vi "AlliGator Update Settings & Control.vi"(7 "Control Label":string, 8 "Error In":errorcluster, 9 "Value":variant, 10 "Sender":string="AlliGator", 11 "CtlRef":refnum<vi>) -> (0 "Error Out":errorcluster)   [LabVIEW 2021, in "AlliGator Settings.lvlib"]
doc: "Updates the Control whose reference or label is passed.\nThe Settings window is updated as well (or if the Settings Window is the sender, AlliGator is)."
uses:
  AlliGator Settings.lvlib
  AlliGator Settings Event.ctl
  AlliGator Settings Window Messages.ctl
  AlliGator Settings List.ctl
  <vilib>/Utility/error.llb/Error Cluster From Error Code.vi
  Variant/Variant to Data/Variant to Boolean.vi
  <vilib>/ErrorRing/Error Ring.xnode
  Variant/Variant to Data/Variant to Data.lvlib
  Notebook/Notebook.lvlib
  Rich Text Box/Rich Text Box.lvlib
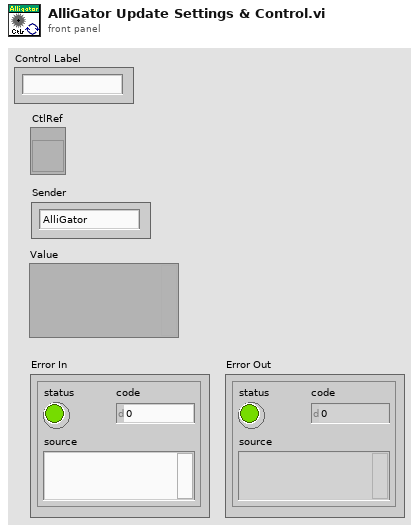
[diagram p1: front panel]
types:
  T1 = typedef "AlliGator Settings.lvlib/AlliGator Settings List.ctl" = enum16{"GUI:Visible Settings Tab", "GUI:Last Run Version", "Source Image:Use Image Histogram for Contrast", "Source Image:Low Count Pixels Rejection Options", "Source Image:High Count Pixels Rejection Options", "Source Image:Use Image Brightness", "Source Image:Blend Overlay with Image Background", "Source Image:Use Fixed ROI Diameter", "Source Image:ROI Diameter", "Source Image:ROI Center Color", "Source Image:Peak Threshold", "Source Image:Intensity Threshold", "Source Image:Image Binning Options", "Source Image:Image Smoothing Options", "Source Image:Image Histogram Active", "Source Image:Invert Binary Mask", "Source Image:Hot Pixel Removal", "Source Image:Overlay Analyzed ROI Center", "Source Image:Auto-Adjust Contrast", "Source Image:Histogram Lower Percentile", "Source Image:Histogram Upper Percentile", "Source Image:Save Source Image", "Source Image:Scale Bar Options", "Source Image:Image Resolution (Pixel Size)", "Source Image:Flatfield Correction", "Source Image:Show Dead Left Columns Correction", "Source Image:Dead Left Columns Correction", "Source Image:Image Pre-Processing Operations Order", "Source Image:Overlay ROI Median", "Source Image:Median Overlay Color", "Data Information:Gate Width", "Data Information:Nanotime Gate Separation", "Data Information:Macrotime Gate Separation", "Data Information:Gate Step", "Data Information:# Gates", "Data Information:Gate Image Exposure", "Data Information:Gate Image Integration", "Data Information:Gates to Skip", "Data Information:Gates to Keep", "Data Information:Define Gates to", "Data Information:Channel Name", "Data Information:Available Channel Names", "Data Information:Channel Arithmetic", "Data Information:Background File Subtraction", "Data Information:Background File", "Data Information:Background Scaling Factor", "Data Information:Background Pile-up Correction", "Data Information:Background Pixel Well Capacity", "Data Information:Laser Period", "Data Information:SYNC Period", "Data Information:Pile-up Correction", "Data Information:Pixel Well Capacity", "Data Information:Dataset Scaling Factor", "Fluorescence Decay_Decay Pre-Processing:Reverse Gates", "Fluorescence Decay_Decay Pre-Processing:Verbose Decay Pre-Processing", "Fluorescence Decay_Decay Pre-Processing:Use Decay Pre-Processing", "Fluorescence Decay_Decay Pre-Processing:Background Subtraction", "Fluorescence Decay_Decay Pre-Processing:Background Definition Range", "Fluorescence Decay_Decay Pre-Processing:Baseline Subtraction Method", "Fluorescence Decay_Decay Pre-Processing:Decay Pre-Processing Operations Order", "Fluorescence Decay_Decay Pre-Processing:Smoothing Parameter", "Fluorescence Decay_Decay Pre-Processing:Shift Decay", "Fluorescence Decay_Decay Pre-Processing:Decay Shift Parameters", "Fluorescence Decay_Decay Pre-Processing:Fold Decay", "Fluorescence Decay_Decay Pre-Processing:# Folds", "Fluorescence Decay_Decay Pre-Processing:1-Normalize Decay", "Fluorescence Decay_Decay Pre-Processing:[0-1]-Normalize Decay", "Fluorescence Decay_Decay Pre-Processing:Smoothen Decay", "Fluorescence Decay_Decay Pre-Processing:Extrapolate Decay", "Fluorescence Decay_Decay Pre-Processing:Use Periodicity", "Fluorescence Decay_Decay Pre-Processing:Use Cursors", "Fluorescence Decay_Decay Pre-Processing:Tail Fraction", "Fluorescence Decay_Decay Pre-Processing:Head Fraction", "Fluorescence Decay_Decay Pre-Processing:Additional Points", "Fluorescence Decay_Decay Pre-Processing:Straighten Decay", "Fluorescence Decay_Decay Pre-Processing:Constant Background", "Fluorescence Decay_Decay Pre-Processing:Pixel-Normalize Decay", "Fluorescence Decay_Advanced Analysis:Extract IRF instead of Decay", "Fluorescence Decay_Advanced Analysis:IRF Extraction Options", "Fluorescence Decay_Advanced Analysis:IRF Optimization Options", "Fluorescence Decay_Advanced Analysis:Square Pulse Options", "Fluorescence Decay_Advanced Analysis:IRF Order", "Fluorescence Decay_Advanced Analysis:IRF Time Constants", "Fluorescence Decay_Advanced Analysis:Wavelet Analysis Options", "Fluorescence Decay_Advanced Analysis:Average Lifetime Options", "Fluorescence Decay_Fit Options:Fit Options", "Fluorescence Decay_Fit Options:Use Legacy Fitting Approach", "Fluorescence Decay_Fit Options:Use Data Information Laser Period", "Fluorescence Decay_Fit Parameters:Displayed Fit Parameters", "Fluorescence Decay_Fit Parameters:Fit Parameter Constraints", "Fluorescence Decay_Fit Parameters:Export Tabulated Results", "Fluorescence Decay_Fit Parameters:MLE Baseline Offset Type", "Fluorescence Decay_Fit Parameters:MLE Baseline Offset", "Fluorescence Decay_Fit Parameters:Guess Parameter Names", "Fluorescence Decay_Fit Parameters:Guess Parameter Values", "Fluorescence Decay_Fit Parameters:Guess Parameters Options", "Fluorescence Decay_Styles:Show Last Decay Only", "Fluorescence Decay_Styles:Decay Graph Color Array", "Fluorescence Decay:Decay Graph Active", "Fluorescence Decay Statistics:Min Peak Value", "Fluorescence Decay Statistics:Reject Low Decay Peak Pixels", "Fluorescence Decay Statistics:Reject High Decay Peak Pixels", "Fluorescence Decay Statistics:Max Peak Value", "Time Traces:Use File Timestamp", "Time Traces:Time Step", "Time Traces:Use Intensity Correction File", "Time Traces:Intensity Correction File", "Phasor Plot:Phasor Plot Smoothing Options", "Phasor Plot:Phasor Plot Size", "Phasor Plot:Phasor Plot Graphics Options", "Phasor Plot:Cumulative Phasor Plot", "Phasor Plot:Use Phasor Brightness", "Phasor Plot:Blend Overlay with Phasor Background", "Phasor Plot:Save Phasor Plot", "Phasor Plot:Show References", "Phasor Plot:Phasor Ratio Decay Range", "Phasor Plot:Exponential Fading", "Phasor Plot:Phasor Ratio Reference Colors", "Phasor Plot:Reference Radius", "Phasor Plot:Show Color Map Vertices", "Phasor Plot:Phasor Plot Active", "Phasor Plot:Phasor Ratio Color Map Type", "Phasor Plot:Phasor Ratio Color Map", "Phasor Plot:Phasor Ratio Display Range", "Phasor Plot:Selected Image ROI(s)", "Phasor Plot:All Image ROIs", "Phasor Plot:Selected Phasor Plot ROI(s)", "Phasor Plot:All Phasor Plot ROIs", "Phasor Plot:Phasor Ratio Color-Coded Quantity", "Phasor Plot:Store Phasor Harmonics", "Phasor Plot:Draw Reference Segment", "Phasor Plot:User-Defined Quantity", "Phasor Graph:Phasor Frequency", "Phasor Graph:Phasor Ratio Type", "Phasor Graph:Pixel-level Phasor Computation", "Phasor Graph:Save Phasor Graph", "Phasor Graph:Phasor Graph Active", "Phasor Graph:Phasor SDV Options", "Phasor Calibration:Use Backup Calibration if needed", "Phasor Graph:Define Shortest Lifetime as", "Phasor Calibration:Backup Calibration Type", "Phasor Calibration:Calibration Type", "Phasor Calibration:Calibration Lifetime", "Phasor Calibration:Calibration Map Algorithm", "Single-Exponential Phasor Locus (SEPL):Gate Parameters", "Single-Exponential Phasor Locus (SEPL):User-defined Gate", "Single-Exponential Phasor Locus (SEPL):User-defined IRF", "Single-Exponential Phasor Locus (SEPL):Phasor Parameters", "Single-Exponential Phasor Locus (SEPL):Decay & IRF Parameters", "Single-Exponential Phasor Locus (SEPL):Display Parameters", "Lifetime Analysis:Decay Analysis Parameters", "Lifetime Analysis:Lifetime Map Active", "Plugins:Python Settings", "Miscellaneous:Verbose Mode", "Miscellaneous:Beep after Script", "Miscellaneous:Saved Image File Format", "Miscellaneous:Exported Gate Image Settings", "Miscellaneous:Include Loading in Timing", "Miscellaneous:Verbose Settings Mode", "Miscellaneous:Histogram Options", "Miscellaneous:Beep on Error", "Miscellaneous:# Logical Processors Used", "Miscellaneous:ROI Description Max Characters", "Miscellaneous:Verbose Error Mode", "Miscellaneous:Transparent Mask Color"}
  T2 = typedef "AlliGator Settings.lvlib/AlliGator Settings Event.ctl" = cluster{"AlliGator Settings Message":T3, "Sender":string, "Control Label":string, "Data":variant}
  T3 = typedef "AlliGator Settings.lvlib/AlliGator Settings Window Messages.ctl" = enum16{"Idle", "Subscribe", "Unsubscribe", "Refresh Parameter", "Refresh All Parameters", "Quit"}
  T4 = typedef "Rich Text Box.lvlib/Text Formatting.ctl" = cluster{"Font":string, "Text Color":T5, "Text Background Color":T5, "Text Style":enum16{"Regular", "Bold", "Italic", "Underline", "Strikeout"}, "Font Size (Points)":dbl, "Text Alignment":i32}
  T5 = typedef "Rich Text Box.lvlib/Text Colors.ctl" = enum16{"Unchanged", "Black", "Blue", "Brown", "Gray", "Green", "Orange", "Pink", "Red", "White"}
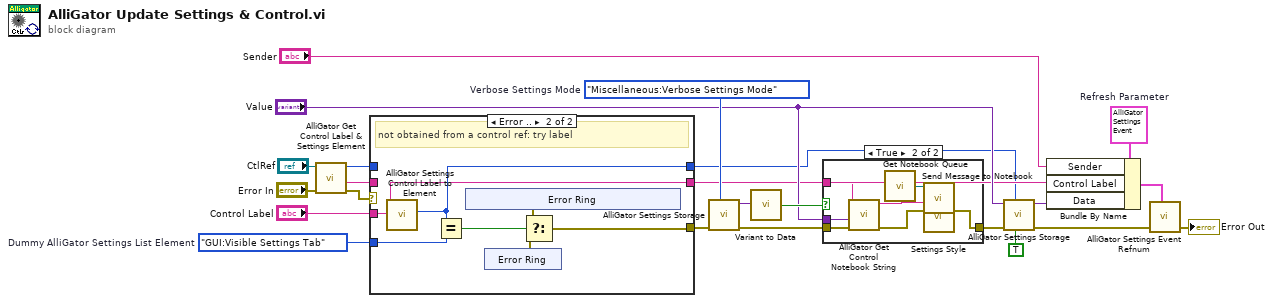
[diagram p0: block diagram]
diagram:
  w2 = AlliGator_Settings_List."GUI:Visible Settings Tab"  # Dummy AlliGator Settings List Element
  w14 = AlliGator_Settings_List."Miscellaneous:Verbose Settings Mode"  # Verbose Settings Mode
  w15 = T2 {"AlliGator Settings Message"=enum."Refresh Parameter", "Sender"="", "Control Label"="", "Data"=variant}  # Refresh Parameter
  n1 = call "AlliGator Get Control Label & Settings Element.vi"("Error In"="Error In", "CtlRef"="CtlRef") -> ("Error Out"=w8:errorcluster, "Control Label"=w6:string, "AlliGator Settings List Element"=w7:T1)  [unwired: 7 in]
  n2 = case shown="Error .." w8 {
    selector: w8 -> [w24 _]
    tunnel: w7 -> [w26 _]
    tunnel: [w26 w33] -> w1
    tunnel: w6 -> [w25 _]
    tunnel: [w25 w28] -> w5
    tunnel: [w24 w29] -> w4
    tunnel: "Control Label" -> [_ w28]
    tunnel: w2 -> [_ w32]
    frame No Error {
      # "valid ontrol reference passed"
    }
    frame Error {
      # "not obtained from a control ref: try label"
      n3 = call "AlliGator Settings Control Label to Element.vi"("Control Label"=w28) -> ("AlliGator Settings List Element"=w33:T1)  [unwired: 7 in, 1 out]
      n4 = Equal?(x=w33, y=w32) -> (x = y?=w31:bool)
      n5 = xnode "Error Ring"() -> ("error out"=w30:errorcluster)
      n6 = xnode "Error Ring"() -> ("error out"=w27:errorcluster)
      n7 = Select(t=w30, s=w31, f=w27) -> (s? t:f=w29:errorcluster)
    }
  }
  n8 = call "AlliGator Settings Storage.vi"("AlliGator Settings List"=w14, "Error In"=w4) -> ("Error Out"=w10:errorcluster, "Variant Data out"=w13:variant)  [unwired: 8 in]
  n9 = call-poly "Variant to Data.vi"("Variant"=w13) -> ("Value"=w12:bool)  [unwired: 8 in]
  n10 = case shown="True" w12 {
    tunnel: w5 -> [_ w47]
    tunnel: "Value" -> [_ w46]
    tunnel: w10 -> [w39 w45]
    tunnel: [w39 w42] -> w9
    frame False {
    }
    frame True {
      n11 = call "AlliGator Get Control Notebook String.vi"("error in (no error)"=w45, "Value"=w46, "Control Label"=w47) -> ("error out"=w41:errorcluster, "Notebook String"=w43:string)  [unwired: 7 in]
      n12 = call "Get Notebook Queue.vi"() -> ("Notebook Queue"=w44:refnum<queue>)  [unwired: 9 in]
      n13 = call "Settings Style.vi"() -> ("Settings Text Formatting"=w40:T4)
      n14 = call "Send Message to Notebook.vi"("Text Formatting"=w40, "Error In"=w41, "Message"=w43, "Notebook Queue"=w44) -> ("Error Out"=w42:errorcluster)  [unwired: 4 in, 1 out]
    }
  }
  n15 = call "AlliGator Settings Storage.vi"("Get(F)/Set"=TRUE, "AlliGator Settings List"=w1, "Error In"=w9, "Variant Data in"="Value") -> ("Error Out"=w18:errorcluster, "Variant Data out"=w19:variant)  [unwired: 6 in]
  n16 = Bundle By Name(cluster=w15, "Sender"="Sender", "Control Label"=w5, "Data"=w19) -> (w16:T2)
  n17 = call "AlliGator Settings Event Refnum.vi"("AlliGator Settings Event"=w16, "Error In"=w18) -> ("Error Out"=→"Error Out":errorcluster)  [unwired: 6 in, 1 out]
